vi "IntraX_.vi"(7 "DeltaE":dbl=1.0 format="%#_13g", 8 "error in (no error)":errorcluster, 11 "Momentum [MeV/C](pixel)":dbl[](array[numeric])) -> (0 "error out":errorcluster, 1 "delta momentum":dbl, 2 "IntraX":i32, 3 "Ramp Pattern":dbl[](array[numeric]))   [LabVIEW 2020]
uses:
  NI_AALBase.lvlib
panel:
  out "x/y":dbl
  out "Momentum [MeV/C](pixel) out":dbl[](array[numeric])
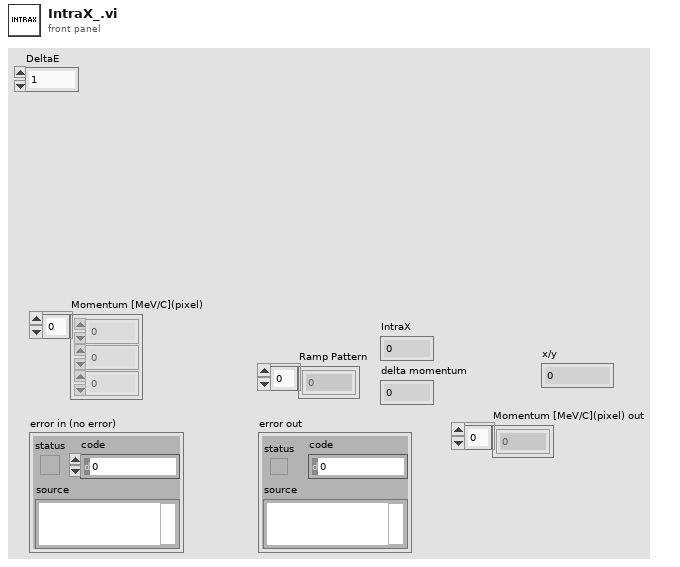
[diagram p1: front panel]
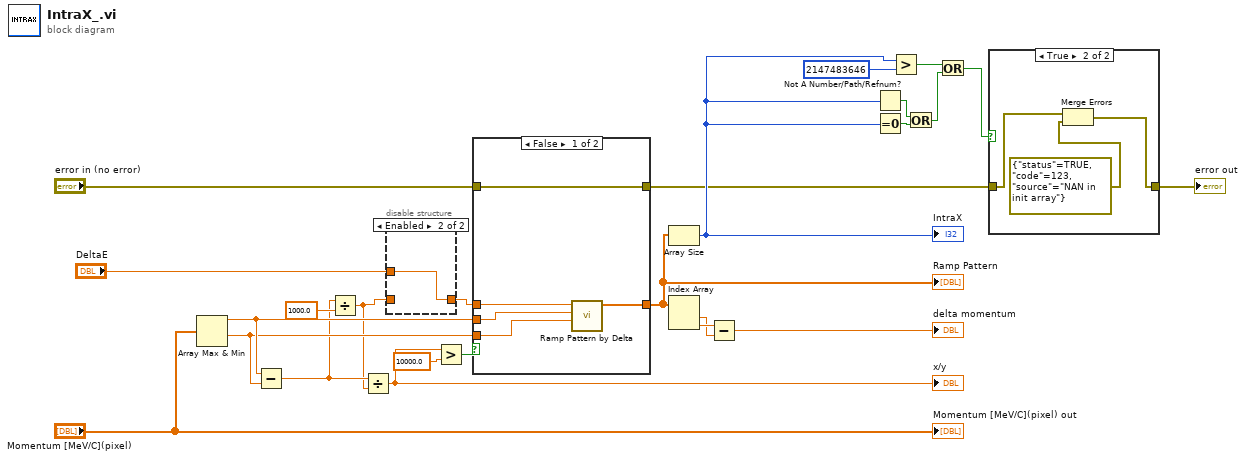
[diagram p0: block diagram]
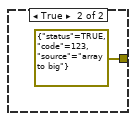
[diagram p4: hidden frame]
diagram:
  n1 = Array Max & Min(array="Momentum [MeV/C](pixel)") -> (max value=w24:dbl, min value=w23:dbl)  [unwired: 2 out]
  n2 = Subtract(x=w24, y=w23) -> (x-y=w6:dbl)
  n3 = Divide(x=w6, y=1000.0) -> (x/y=w3:dbl)
  n4 = Divide(x=w6, y=w3) -> (x/y=w22:dbl)
  "x/y" <- w22
  n5 = disable-structure shown="Enabled" {
    disable-tunnel: w3 -> [w26 _]
    disable-tunnel: [w26 w27] -> w2
    disable-tunnel: "DeltaE" -> [_ w27]
    frame Disabled {
    }
    frame Enabled {
    }
  }
  n6 = Greater?(x=w22, y=10000.0) -> (0:w20:bool)
  n7 = case shown="False" w20 {
    tunnel: [w32 _] -> w16
    tunnel: w24 -> [w31 _]
    tunnel: w23 -> [w30 _]
    tunnel: w2 -> [w29 _]
    tunnel: [w28 errorcluster {"status"=TRUE, "code"=123, "source"="array to big"} ("error in (no error)")] -> w8
    tunnel: "error in (no error)" -> [w28 _]
    frame False {
      n8 = call "Ramp Pattern by Delta.vi"("start"=w30, "end"=w31, "delta"=w29) -> ("Ramp Pattern"=w32:dbl[])  [unwired: 6 in, 2 out]
    }
    frame True {
    }
  }
  "Ramp Pattern" <- w16
  n9 = Array Size(array=w16) -> (size(s)=w9:i32)
  "IntraX" <- w9
  n10 = Index Array(array=w16) -> (element #1=w17:dbl, element #2=w18:dbl)  [unwired: 2 in]
  n11 = Subtract(x=w18, y=w17) -> (x-y=→"delta momentum":dbl)
  n12 = Not A Number/Path/Refnum?(number/path/refnum=w9) -> (NaN/Path/Refnum?=w15:bool)
  n13 = Equal To 0?(x=w9) -> (x = 0?=w14:bool)
  n14 = Greater?(x=w9, y=2147483646) -> (0:w12:bool)
  n15 = Or(x=w15, y=w14) -> (x .or. y?=w11:bool)
  n16 = Or(x=w12, y=w11) -> (x .or. y?=w10:bool)
  n17 = case shown="True" w10 {
    tunnel: w8 -> [w34 w37]
    tunnel: [w34 w35] -> w4
    frame False {
    }
    frame True {
      n18 = Merge Errors(w37, errorcluster {"status"=TRUE, "code"=123, "source"="NAN in init array"} ("error IO")) -> (w35:errorcluster)
    }
  }
  "error out" <- w4
  "Momentum [MeV/C](pixel) out" <- "Momentum [MeV/C](pixel)"
